vi "AlliGator Check Valid Python Plugin Target.vi"(8 "error in (no error)":errorcluster, 9 "Source":string, 11 "Target Found?":bool) -> (0 "error out":errorcluster)   [LabVIEW 2021, in "AlliGator Python Plugins.lvlib"]
doc: "Outputs warning with missing python plugin target."
uses:
  <vilib>/Utility/error.llb/DialogType.ctl
  AlliGator Python Plugins.lvlib
panel:
  # "see the AlliGator License on the block diagram (Ctrl+E or Window:Show Block Diagram)"
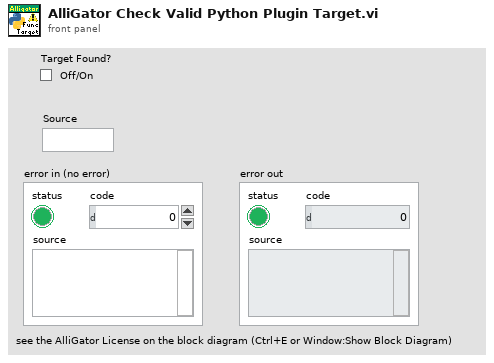
[diagram p1: front panel]
types:
  T1 = typedef "DialogType.ctl" = u16
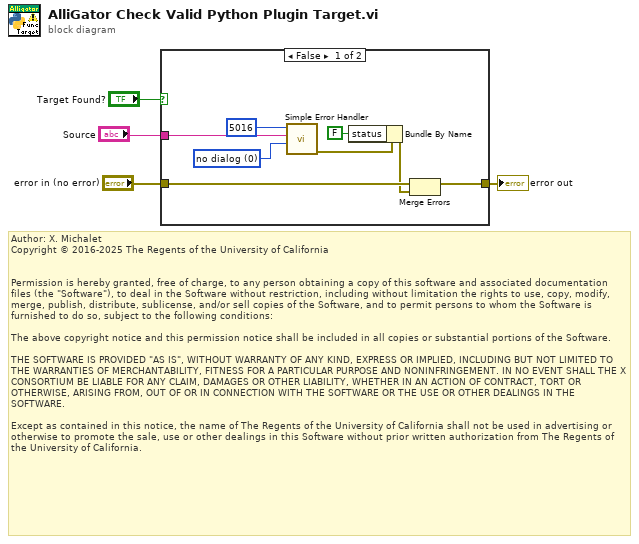
[diagram p0: block diagram]
diagram:
  # "Author: X. Michalet\nCopyright © 2016-2025 The Regents of the University of California\n \n\nPermission is hereby granted, free of charge, to any person obtaining a copy of this software and associated documentation files (the \"Software\"), to deal in the Software without restriction, including without limitation the rights to use, copy, modify, merge, publish, distribute, sublicense, and/or sell copies of the Software, and to permit persons to whom the Software is furnished to do so, subject to the following conditions:\n\nThe above copyright notice and this permission notice shall be included in all copies or substantial portions of the Software.\n\nTHE SOFTWARE IS PROVIDED \"AS IS\", WITHOUT WARRANTY OF ANY KIND, EXPRESS OR IMPLIED, INCLUDING BUT NOT LIMITED TO THE WARRANTIES OF MERCHANTABILITY, FITNESS FOR A PARTICULAR PURPOSE AND NONINFRINGEMENT. IN NO EVENT SHALL THE X CONSORTIUM BE LIABLE FOR ANY CLAIM, DAMAGES OR OTHER LIABILITY, WHETHER IN AN ACTION OF CONTRACT, TORT OR OTHERWISE, ARISING FROM, OUT OF OR IN CONNECTION WITH THE SOFTWARE OR THE USE OR OTHER DEALINGS IN THE SOFTWARE.\n\nExcept as contained in this notice, the name of The Regents of the University of California shall not be used in advertising or otherwise to promote the sale, use or other dealings in this Software without prior written authorization from The Regents of the University of California."
  n1 = case shown="False" "Target Found?" {
    tunnel: [w8 w13] -> w4
    tunnel: "error in (no error)" -> [w7 w13]
    tunnel: "Source" -> [w10 _]
    frame False {
      w9 = T1 0 items=["no dialog", "OK message", "continue or stop message", "OK message + warnings", "continue/stop + warnings"] ("type of dialog (OK msg:1)")
      n2 = call <vilib>:"Simple Error Handler.vi"("error code (no error:0)"=5016, "error source (\" \")"=w10, "type of dialog (OK msg:1)"=w9) -> ("error out"=w12:errorcluster)  [unwired: 2 in, 4 out]
      n3 = Bundle By Name(cluster=w12, "status"=FALSE) -> (w6:errorcluster)
      n4 = Merge Errors(w7, w6) -> (w8:errorcluster)
    }
    frame True {
    }
  }
  "error out" <- w4
